vi "Compute Residuals ACF.vi"(8 "Error In":errorcluster, 11 "Residual Plot in":cluster{"X Array":dbl[], "Y Array":dbl[]}) -> (0 "Error Out":errorcluster, 1 "ACF SDV":dbl, 2 "ACF Mean":dbl, 3 "Residual ACF out":cluster{"X Array":dbl[], "Y Array":dbl[]}, 4 "ACF Statistics":string)   [LabVIEW 2021, in "Fits.lvlib"]
uses:
  Fits.lvlib
  <vilib>/Analysis/2dsp.llb/1D Auto Correlation (DBL).vi
  9a873d00-1c09-4617-ba10-345cef13fe89.vi
  <vilib>/Utility/error.llb/Error Cluster From Error Code.vi
  <vilib>/Analysis/NI_AALPro.lvlib
  Error/Error.lvlib
panel:
  # "see the License on the block diagram (Ctrl+E or Window:Show Block Diagram)"
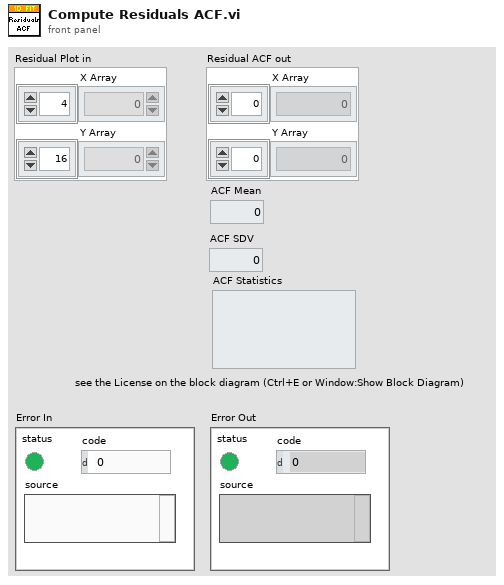
[diagram p1: front panel]
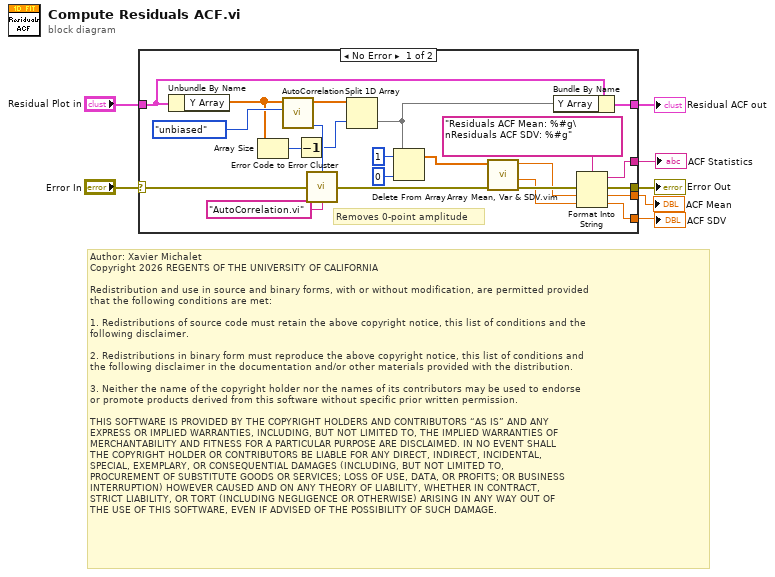
[diagram p0: block diagram]
diagram:
  # "Author: Xavier Michalet\nCopyright 2026 REGENTS OF THE UNIVERSITY OF CALIFORNIA\n\nRedistribution and use in source and binary forms, with or without modification, are permitted provided\nthat the following conditions are met:\n\n1. Redistributions of source code must retain the above copyright notice, this list of conditions and the\nfollowing disclaimer.\n\n2. Redistributions in binary form must reproduce the above copyright notice, this list of conditions and\nthe following disclaimer in the documentation and/or other materials provided with the distribution.\n\n3. Neither the name of the copyright holder nor the names of its contributors may be used to endorse \nor promote products derived from this software without specific prior written permission.\n\nTHIS SOFTWARE IS PROVIDED BY THE COPYRIGHT HOLDERS AND CONTRIBUTORS “AS IS” AND ANY \nEXPRESS OR IMPLIED WARRANTIES, INCLUDING, BUT NOT LIMITED TO, THE IMPLIED WARRANTIES OF\nMERCHANTABILITY AND FITNESS FOR A PARTICULAR PURPOSE ARE DISCLAIMED. IN NO EVENT SHALL\nTHE COPYRIGHT HOLDER OR CONTRIBUTORS BE LIABLE FOR ANY DIRECT, INDIRECT, INCIDENTAL, \nSPECIAL, EXEMPLARY, OR CONSEQUENTIAL DAMAGES (INCLUDING, BUT NOT LIMITED TO, \nPROCUREMENT OF SUBSTITUTE GOODS OR SERVICES; LOSS OF USE, DATA, OR PROFITS; OR BUSINESS\nINTERRUPTION) HOWEVER CAUSED AND ON ANY THEORY OF LIABILITY, WHETHER IN CONTRACT, \nSTRICT LIABILITY, OR TORT (INCLUDING NEGLIGENCE OR OTHERWISE) ARISING IN ANY WAY OUT OF\nTHE USE OF THIS SOFTWARE, EVEN IF ADVISED OF THE POSSIBILITY OF SUCH DAMAGE."
  n1 = case shown="No Error" "Error In" {
    selector: "Error In" -> [w28 w30]
    tunnel: [w16 w30] -> w6
    tunnel: "Residual Plot in" -> [w23 w29]
    tunnel: [w22 w29] -> w4
    tunnel: [w14 _] -> w3
    tunnel: [w13 _] -> w2
    tunnel: [w12 _] -> w1
    frame No Error {
      # "Removes 0-point amplitude"
      n2 = Unbundle By Name(w23) -> ("Y Array"=w21:dbl[])
      n3 = Array Size(array=w21) -> (size(s)=w20:i32)
      n4 = call-poly <vilib>:"AutoCorrelation.vi"("normalization"=enum32{"none", "unbiased", "biased"}."unbiased", "X"=w21) -> ("error"=w26:i32, "Rxx"=w24:dbl[])  [unwired: 8 in]
      n5 = Decrement(x=w20) -> (x-1=w11:i32)
      n6 = call "Error Code to Error Cluster.vi"("Error Code"=w26, "Error Source"="AutoCorrelation.vi", "Error In"=w28) -> ("Error Out"=w18:errorcluster)  [unwired: 12 in]
      n7 = Split 1D Array(array=w24, index=w11) -> (second subarray=w19:dbl[])  [unwired: 1 out]
      n8 = Delete From Array(array=w19, length=1, index=0) -> (array with subset deleted=w10:dbl[])  [unwired: 1 out]
      n9 = call "Array Mean, Var & SDV.vim"("Error In"=w18, "Array"=w10) -> ("Error Out"=w17:errorcluster, "Array SDV"=w12:dbl, "Array Mean"=w13:dbl)  [unwired: 4 in, 3 out]
      n10 = Bundle By Name(cluster=w23, "Y Array"=w19) -> (w22:cluster{"X Array":dbl[], "Y Array":dbl[]})
      n11 = Format Into String(format string="Residuals ACF Mean: %#g\nResiduals ACF SDV: %#g", error in=w17, w13, w12) -> (resulting string=w14:string, error out=w16:errorcluster)  [unwired: 1 in]
    }
    frame Error {
    }
  }
  "Residual ACF out" <- w4
  "Error Out" <- w6
  "ACF Statistics" <- w3
  "ACF Mean" <- w2
  "ACF SDV" <- w1
